vi "DAQmx_Analogue_Measurement_length_check.vi"(9 "Input ranges in":dbl[](array[numeric]), 10 "Requested length":i32) -> (3 "Input ranges out":dbl[](array[numeric]))   [LabVIEW 2016]
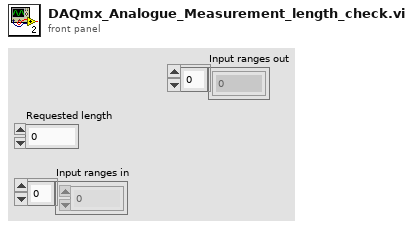
[diagram p1: front panel]
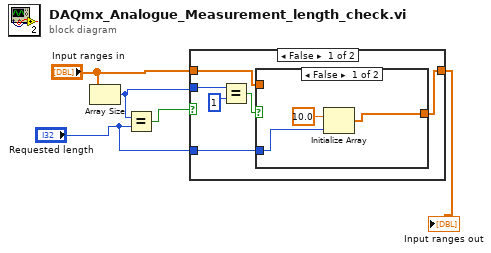
[diagram p0: block diagram]
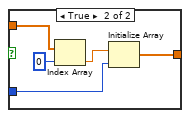
[diagram p2: hidden frame]
diagram:
  n1 = Array Size(array="Input ranges in") -> (size(s)=w1:i32)
  n2 = Equal?(x=w1, y="Requested length") -> (x = y?=w3:bool)
  n3 = case shown="False" w3 {
    tunnel: [w6 w20] -> w4
    tunnel: "Input ranges in" -> [w8 w20]
    tunnel: w1 -> [w11 _]
    tunnel: "Requested length" -> [w7 _]
    frame False {
      n4 = Equal?(x=w11, y=1) -> (x = y?=w9:bool)
      n5 = case shown="False" w9 {
        tunnel: w8 -> [_ w18]
        tunnel: w7 -> [w14 w16]
        tunnel: [w12 w15] -> w6
        frame False {
          n6 = Initialize Array(10.0 ("element"), w14) -> (w12:dbl[])
        }
        frame True {
          n7 = Index Array(array=w18, index=0) -> (element=w17:dbl)
          n8 = Initialize Array(w17, w16) -> (w15:dbl[])
        }
      }
    }
    frame True {
    }
  }
  "Input ranges out" <- w4
